vi "Circular Buffer(2D Wfm with Attributes).vi"(7 "Buffer Size":T3, 8 "error in (no error)":errorcluster, 9 "Read Size":i32, 10 "Operation":T1, 11 "Data In":waveform(dbl)[](array[waveform])) -> (0 "error out":errorcluster, 1 "Elements Remaining":i32, 2 "Buffer Status":T2, 3 "Data Out":waveform(dbl)[](array[waveform]))   [LabVIEW 2016, in "Circular Buffer.lvlib"]
doc: "This VI implements a circular buffer which data can be written to and read from. There can only be one buffer per data type at once, but you can have multiple buffers of different types at the same time. For example, you can have a buffer of Wfm data types as well as I32s in the same VI. You cannot have two independent buffers of I32s."
uses:
  Circular Buffer.lvlib
  Controls/Circular Buffer Status.ctl
  Controls/Circular Buffer Operations.ctl
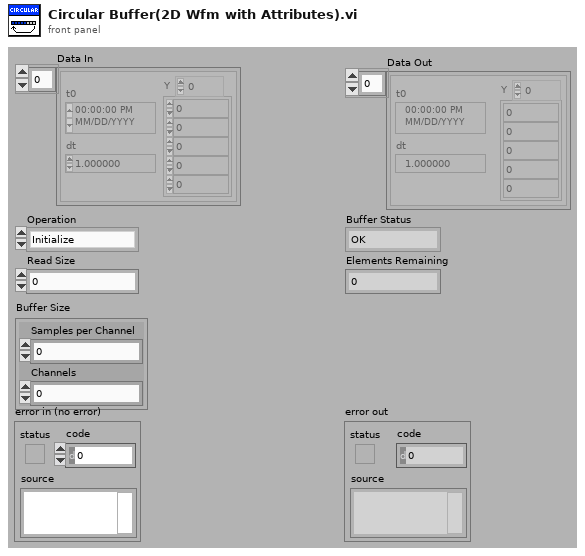
[diagram p1: front panel]
types:
  T1 = typedef "Circular Buffer.lvlib/Circular Buffer Operations.ctl" = enum16{"Initialize", "Get Backlog", "Write", "Read (continuous)", "Read (most recent)"}
  T2 = typedef "Circular Buffer.lvlib/Circular Buffer Status.ctl" = enum16{"OK", "Overflow", "Underflow"}
  T3 = cluster{"Samples per Channel":u32, "Channels":u32}
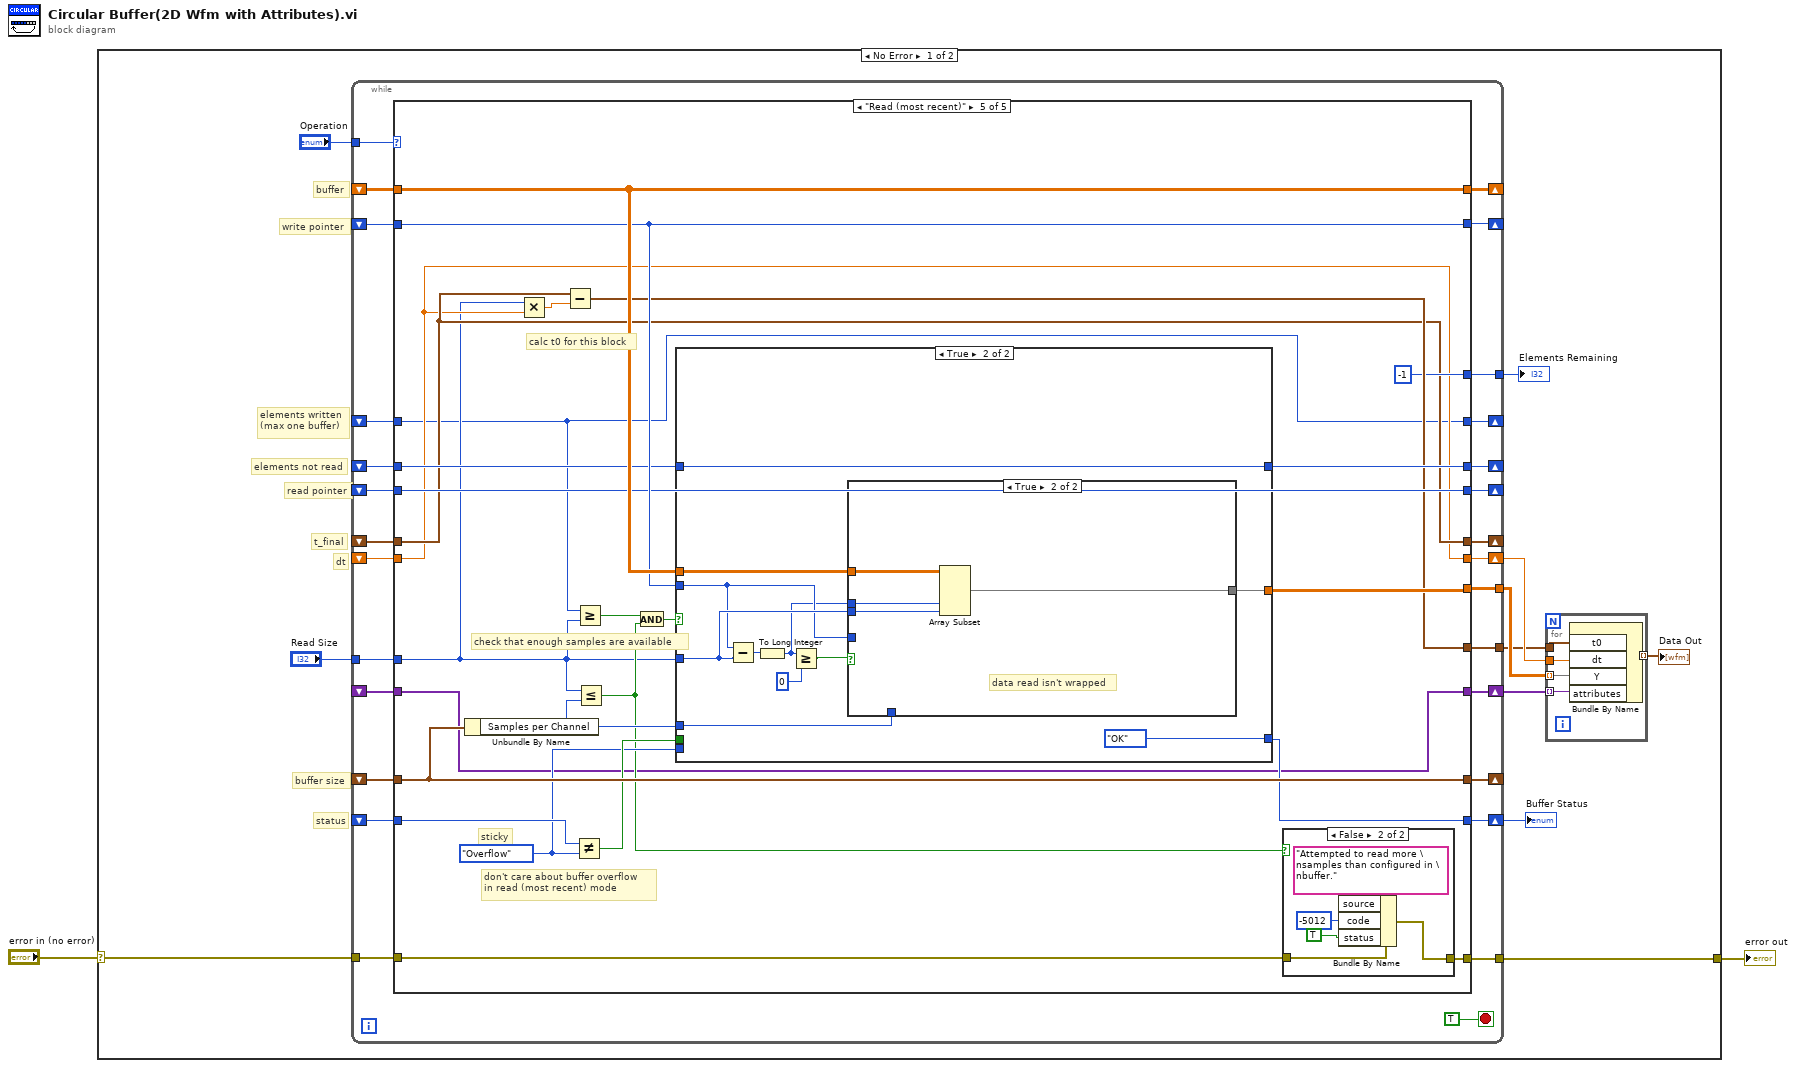
[diagram p0: block diagram]
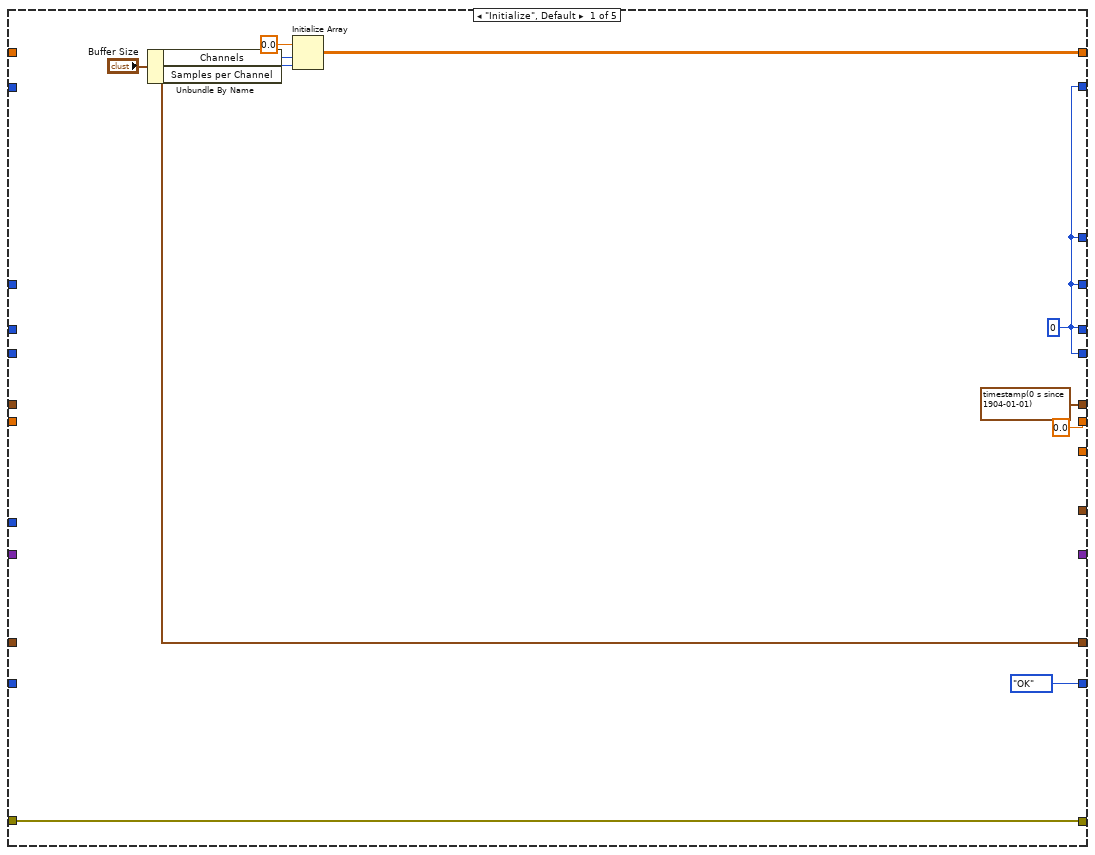
[diagram p2: hidden frame]
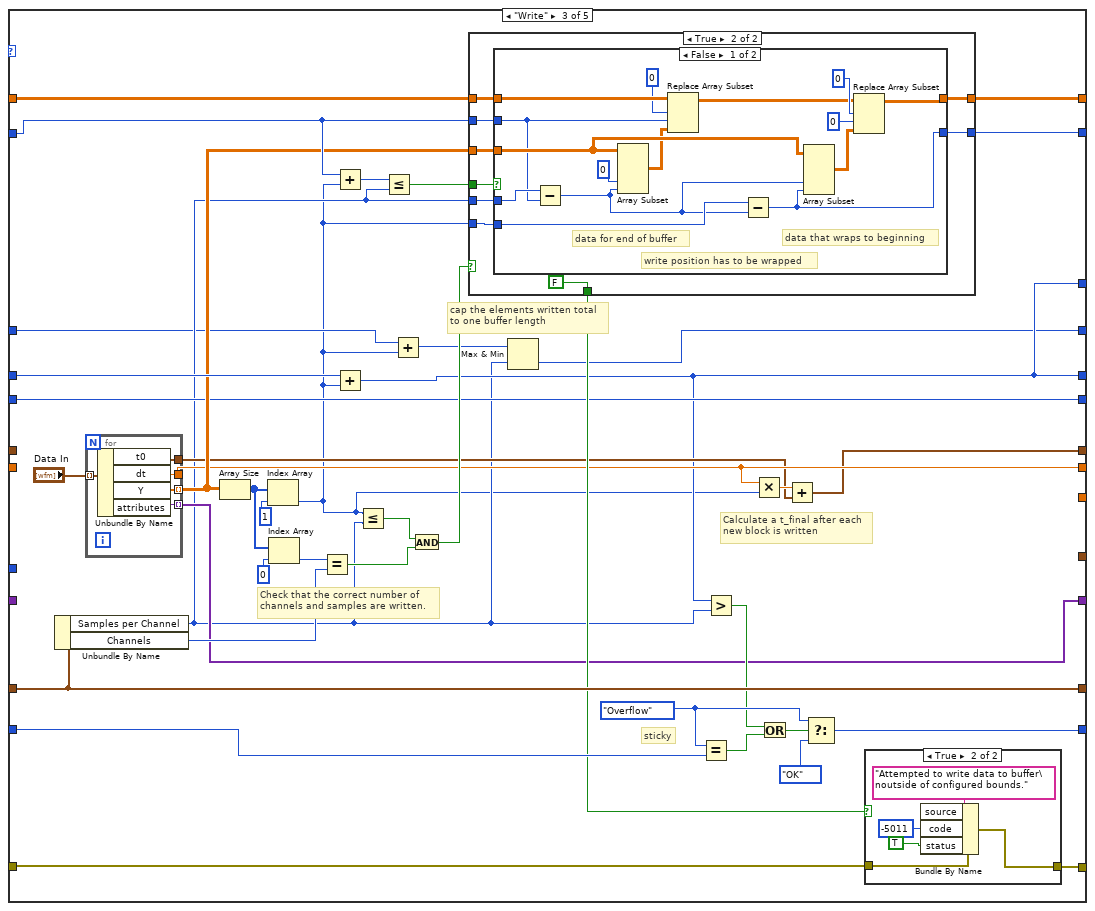
[diagram p4: hidden frame]
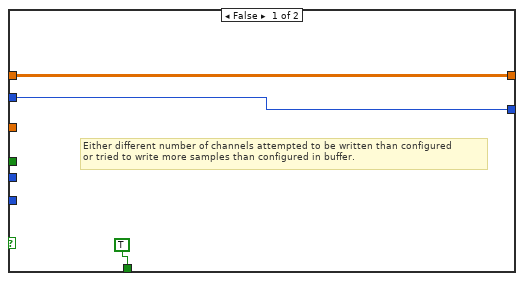
[diagram p6: hidden frame]
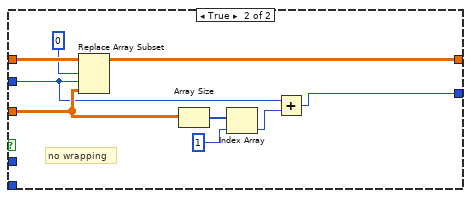
[diagram p7: hidden frame]
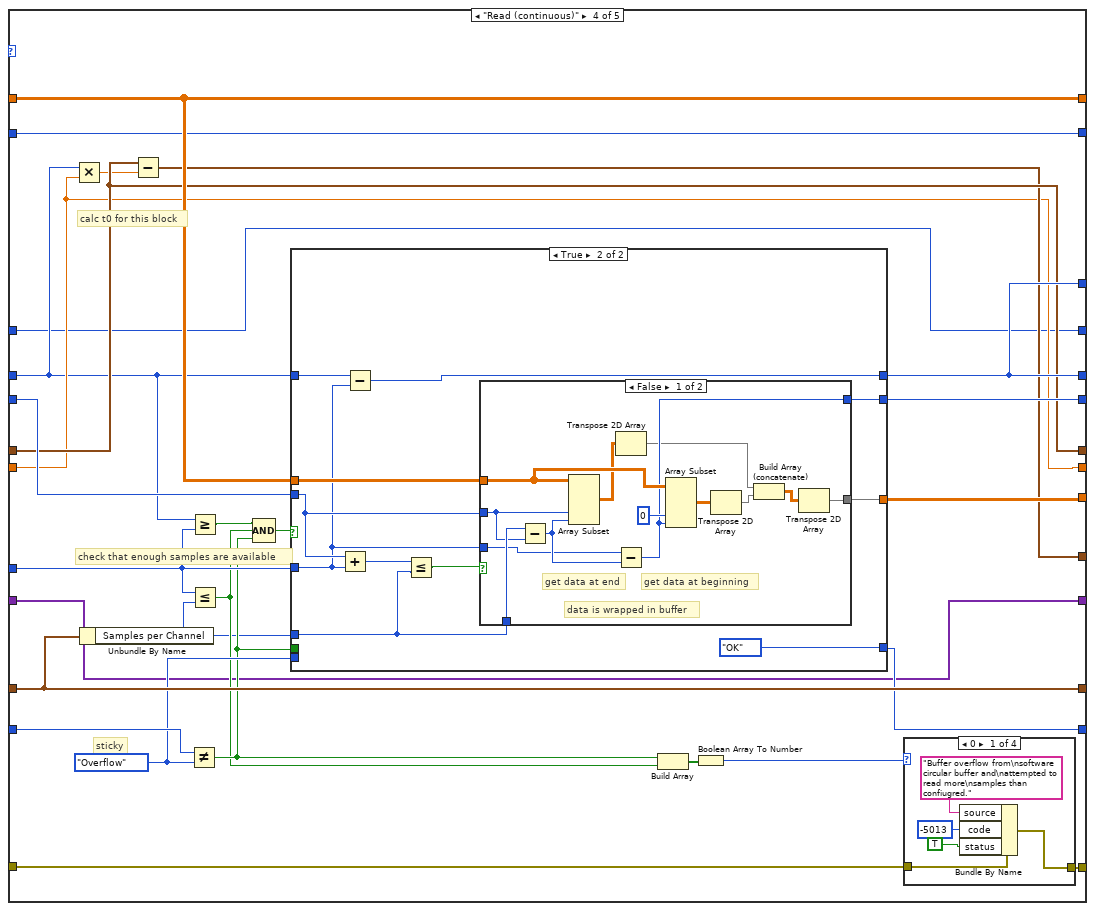
[diagram p8: hidden frame]
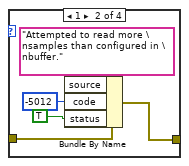
[diagram p9: hidden frame]
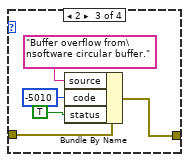
[diagram p10: hidden frame]
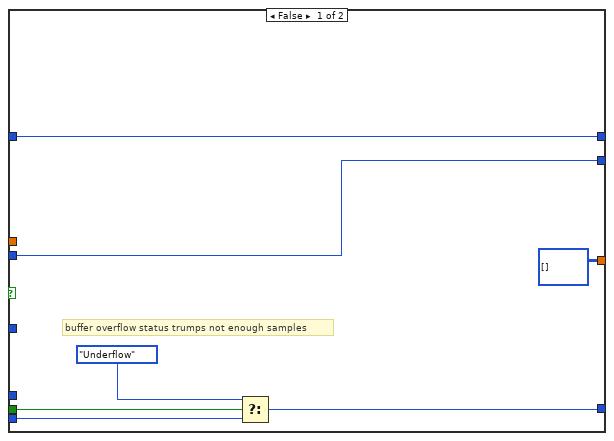
[diagram p12: hidden frame]
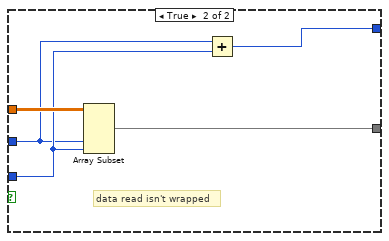
[diagram p13: hidden frame]
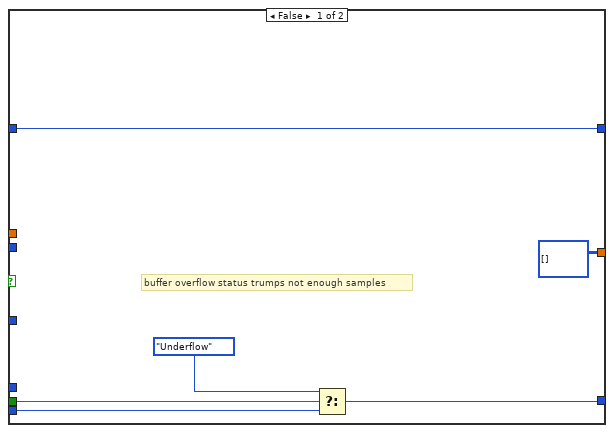
[diagram p15: hidden frame]
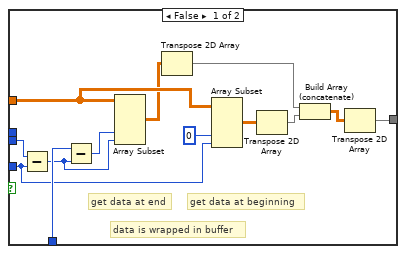
[diagram p16: hidden frame]
diagram:
  n1 = case shown="No Error" "error in (no error)" {
    selector: "error in (no error)" -> [w10 w298]
    tunnel: [w9 w298] -> w1
    frame No Error {
      # "elements written\n(max one buffer)"
      # "dt"
      # "t_final"
      # "write pointer"
      # "status"
      # "buffer size"
      # "read pointer"
      # "elements not read"
      # "buffer"
      n2 = while {
        tunnel: "Operation" -> [w45]
        shift-right: [w44] -> _
        shift-left: _ -> [w41]
        shift-right: [w43] -> _
        shift-left: _ -> [w40]
        shift-right: [w42] -> _
        shift-left: _ -> [w37]
        shift-right: [w39] -> _
        shift-left: _ -> [w38]
        tunnel: "Read Size" -> [w36]
        shift-right: [w35] -> w12
        shift-left: _ -> [w34]
        tunnel: [w33] -> w7
        tunnel: [w32] -> w9
        tunnel: w10 -> [w31]
        shift-right: [w30] -> _
        shift-left: _ -> [w29]
        shift-right: [w28] -> _
        shift-left: _ -> [w26]
        shift-right: [w27] -> w6
        shift-left: _ -> [w25]
        tunnel: [w24] -> w5
        tunnel: [w23] -> w4
        shift-right: [w22] -> w3
        shift-left: _ -> [w21]
        shift-right: [w19] -> _
        shift-left: _ -> [w20]
        stop <- TRUE stop-if-true
        n3 = case shown="\"Read (most recent)\"" w45 {
          tunnel: [w55 w65 w83 w180 w257] -> w44
          tunnel: [w47 w58 w71 w161 w252] -> w43
          tunnel: [w47 w60 w78 w163 w248] -> w42
          tunnel: w41 -> [_ w65 w82 w180 w257]
          tunnel: w40 -> [_ w58 w97 w156 w239]
          tunnel: ["Buffer Size" w59 w106 w179 w256] -> w39
          tunnel: w38 -> [_ w59 w106 w179 w256]
          tunnel: w37 -> [_ w60 w78 w176 w248]
          tunnel: w36 -> [_ _ _ w171 w236]
          tunnel: [Circular_Buffer_Status."OK" ("status") w64 w105 w175 w251] -> w35
          tunnel: w34 -> [_ w64 w102 w178 w255]
          tunnel: [_ _ _ w172 w250] -> w33
          tunnel: [w50 w66 w91 w174 w246] -> w32
          tunnel: w31 -> [w50 w66 w90 w173 w247]
          tunnel: [w47 w61 w79 w164 w249] -> w30
          tunnel: w29 -> [_ w61 w94 w164 w249]
          tunnel: [timestamp(0 s since 1904-01-01) ("t0") w63 w74 w160 w238] -> w28
          tunnel: [0.0 ("dt") w62 w76 w157 w237] -> w27
          tunnel: w26 -> [_ w63 _ w160 w238]
          tunnel: w25 -> [_ w62 _ w157 w237]
          tunnel: [_ _ _ w159 w241] -> w24
          tunnel: [w47 w58 w71 w161 -1] -> w23
          tunnel: [_ _ w73 w155 w234] -> w22
          tunnel: w21 -> [_ _ _ w155 w234]
          tunnel: w20 -> [_ w57 w69 w154 w233]
          tunnel: [w47 w57 w68 w154 w233] -> w19
          frame "Initialize", Default {
            w47 = 0 ("dimension size 2")
            n4 = Unbundle By Name("Buffer Size") -> ("Channels"=w52:u32, "Samples per Channel"=w51:u32)
            n5 = Initialize Array(0.0 ("element"), w52, w51) -> (w55:dbl[][])
          }
          frame "Get Backlog" {
          }
          frame "Write" {
            w101 = Circular_Buffer_Status."Overflow" ("status")
            # "cap the elements written total\nto one buffer length"
            # "Calculate a t_final after each\nnew block is written"
            # "Check that the correct number of\nchannels and samples are written."
            # "sticky"
            n6 = Unbundle By Name(w106) -> ("Samples per Channel"=w70:u32, "Channels"=w87:u32)
            n7 = for {
              tunnel: "Data In" -> [w111] mode=indexing
              tunnel: [w110] -> w80 mode=indexing
              tunnel: [w109] -> w76
              tunnel: [w108] -> w75
              tunnel: [w107] -> w73 mode=indexing
              n8 = Unbundle By Name(w111) -> ("t0"=w108:timestamp, "dt"=w109:dbl, "Y"=w110:dbl[], "attributes"=w107:variant)
            }
            n9 = Array Size(array=w80) -> (size(s)=w93:i32[])
            n10 = Index Array(array=w93, index=1) -> (element=w67:i32)
            n11 = Index Array(array=w93, index=0) -> (element=w88:i32)
            n12 = Equal?(x=w88, y=w87) -> (x = y?=w85:bool)
            n13 = Add(x=w94, y=w67) -> (x+y=w96:u32)
            n14 = Add(x=w97, y=w67) -> (x+y=w71:i32)
            n15 = Less Or Equal?(x=w67, y=w70) -> (x <= y?=w86:bool)
            n16 = Less Or Equal?(x=w96, y=w70) -> (x <= y?=w95:bool)
            n17 = Add(x=w69, y=w67) -> (x+y=w72:u32)
            n18 = And(x=w86, y=w85) -> (x .and. y?=w84:bool)
            n19 = case shown="True" w84 {
              tunnel: [w120 w129] -> w83
              tunnel: w95 -> [_ w128]
              tunnel: [w119 w127] -> w79
              tunnel: w94 -> [w119 w126]
              tunnel: w82 -> [w120 w125]
              tunnel: w80 -> [_ w124]
              tunnel: w67 -> [_ w123]
              tunnel: w70 -> [_ w122]
              tunnel: [TRUE FALSE] -> w89
              frame False {
                # "Either different number of channels attempted to be written than configured\nor tried to write more samples than configured in buffer."
              }
              frame True {
                n20 = case shown="False" w128 {
                  tunnel: w125 -> [w144 w153]
                  tunnel: [w139 w151] -> w129
                  tunnel: w126 -> [w133 w146]
                  tunnel: w124 -> [w137 w148]
                  tunnel: w122 -> [w134 _]
                  tunnel: w123 -> [w136 _]
                  tunnel: [w135 w145] -> w127
                  frame False {
                    # "data that wraps to beginning"
                    # "data for end of buffer"
                    # "write position has to be wrapped"
                    n21 = Subtract(x=w134, y=w133) -> (x-y=w132:u32)
                    n22 = Array Subset(array=w137, index (col)=0 ("index"), length (col)=w132) -> (w131:dbl[][])  [unwired: 2 in]
                    n23 = Replace Array Subset(array=w144, new element=w131, index (row)=0, index (col)=w133) -> (w140:dbl[][])
                    n24 = Subtract(x=w136, y=w132) -> (x-y=w135:u32)
                    n25 = Array Subset(array=w137, index (col)=w132, length (col)=w135) -> (w142:dbl[][])  [unwired: 2 in]
                    n26 = Replace Array Subset(array=w140, new element=w142, index (row)=0, index (col)=0 ("disabled index (col)")) -> (w139:dbl[][])
                  }
                  frame True {
                    # "no wrapping"
                    n27 = Replace Array Subset(array=w153, new element=w148, index (row)=0 ("disabled index (col)"), index (col)=w146) -> (w151:dbl[][])
                    n28 = Array Size(array=w148) -> (size(s)=w150:i32[])
                    n29 = Index Array(array=w150, index=1) -> (element=w147:i32)
                    n30 = Add(x=w146, y=w147) -> (x+y=w145:u32)
                  }
                }
              }
            }
            n31 = Max & Min(x=w72, y=w70) -> (min(x,y)=w68:u32)  [unwired: 1 out]
            n32 = Equal?(x=w101, y=w102) -> (x = y?=w104:bool)
            n33 = Greater?(x=w71, y=w70) -> (0:w99:bool)
            n34 = Multiply(x=w76, y=w67) -> (x*y=w77:dbl)
            n35 = Or(x=w99, y=w104) -> (x .or. y?=w103:bool)
            n36 = Add(x=w77, y=w75) -> (x+y=w74:timestamp)
            n37 = Select(t=w101, s=w103, f=Circular_Buffer_Status."OK" ("status")) -> (s? t:f=w105:T2)
            n38 = case shown="True" w89 {
              tunnel: w90 -> [w112 w117]
              tunnel: [w112 w116] -> w91
              frame False {
              }
              frame True {
                n39 = Bundle By Name(cluster=w117, "source"="Attempted to write data to buffer\noutside of configured bounds.", "code"=-5011, "status"=TRUE) -> (w116:errorcluster)
              }
            }
          }
          frame "Read (continuous)" {
            w177 = Circular_Buffer_Status."Overflow" ("status")
            # "calc t0 for this block"
            # "check that enough samples are available"
            # "sticky"
            n40 = Multiply(x=w156, y=w157) -> (x*y=w158:dbl)
            n41 = Unbundle By Name(w179) -> ("Samples per Channel"=w162:u32)
            n42 = Subtract(x=w160, y=w158) -> (x-y=w159:timestamp)
            n43 = Not Equal?(x=w178, y=w177) -> (x != y?=w168:bool)
            n44 = Greater Or Equal?(x=w156, y=w171) -> (x >= y?=w170:bool)
            n45 = Less Or Equal?(x=w171, y=w162) -> (x <= y?=w167:bool)
            n46 = Compound Arithmetic op=AND(w170, w167, w168) -> (w169:bool)
            n47 = case shown="True" w169 {
              tunnel: w176 -> [w198 w207]
              tunnel: w180 -> [_ w213]
              tunnel: w171 -> [_ w205]
              tunnel: w162 -> [_ w208]
              tunnel: [w202 Circular_Buffer_Status."OK" ("status")] -> w175
              tunnel: w168 -> [w203 _]
              tunnel: w177 -> [w201 _]
              tunnel: w156 -> [w199 w206]
              tunnel: [w199 w204] -> w161
              tunnel: [w198 w209] -> w163
              tunnel: [i32[][] [] w210] -> w172
              frame False {
                # "buffer overflow status trumps not enough samples"
                n48 = Select(t=Circular_Buffer_Status."Underflow" ("status"), s=w203, f=w201) -> (s? t:f=w202:T2)
              }
              frame True {
                n49 = Add(x=w207, y=w205) -> (x+y=w212:u32)
                n50 = Subtract(x=w206, y=w205) -> (x-y=w204:i32)
                n51 = Less Or Equal?(x=w212, y=w208) -> (x <= y?=w211:bool)
                n52 = case shown="False" w211 {
                  tunnel: w213 -> [w226 w232]
                  tunnel: w207 -> [w222 w229]
                  tunnel: w205 -> [w215 w230]
                  tunnel: [w217 w231] -> w210
                  tunnel: [w223 w228] -> w209
                  tunnel: w208 -> [w227 _]
                  frame False {
                    # "get data at beginning"
                    # "get data at end"
                    # "data is wrapped in buffer"
                    n53 = Subtract(x=w227, y=w222) -> (x-y=w224:u32)
                    n54 = Array Subset(array=w226, index (col)=w222, length (col)=w224) -> (w221:dbl[][])  [unwired: 2 in]
                    n55 = Transpose 2D Array(2D array=w221) -> (transposed array=w219:dbl[][])
                    n56 = Subtract(x=w215, y=w224) -> (x-y=w223:u32)
                    n57 = Array Subset(array=w226, index (col)=0 ("index"), length (col)=w223) -> (w220:dbl[][])  [unwired: 2 in]
                    n58 = Transpose 2D Array(2D array=w220) -> (transposed array=w218:dbl[][])
                    n59 = Build Array (concatenate)(w219, w218) -> (w216:dbl[][])
                    n60 = Transpose 2D Array(2D array=w216) -> (transposed array=w217:dbl[][])
                  }
                  frame True {
                    # "data read isn't wrapped"
                    n61 = Array Subset(array=w232, index (col)=w229, length (col)=w230) -> (w231:dbl[][])  [unwired: 2 in]
                    n62 = Add(x=w229, y=w230) -> (x+y=w228:u32)
                  }
                }
              }
            }
            n63 = Build Array(w168, w167) -> (w166:bool[])
            n64 = Boolean Array To Number(Boolean array=w166) -> (number=w165:u32)
            n65 = case shown="0" w165 {
              tunnel: w173 -> [w185 w190 w195 w196]
              tunnel: [w184 w189 w194 w196] -> w174
              frame 0 {
                n66 = Bundle By Name(cluster=w185, "source"="Buffer overflow from\nsoftware circular buffer and\nattempted to read more\nsamples than confiugred.", "code"=-5013, "status"=TRUE) -> (w184:errorcluster)
              }
              frame 1 {
                n67 = Bundle By Name(cluster=w190, "source"="Attempted to read more \nsamples than configured in \nbuffer.", "code"=-5012, "status"=TRUE) -> (w189:errorcluster)
              }
              frame 2 {
                n68 = Bundle By Name(cluster=w195, "source"="Buffer overflow from\nsoftware circular buffer.", "code"=-5010, "status"=TRUE) -> (w194:errorcluster)
              }
              frame 3, Default {
              }
            }
          }
          frame "Read (most recent)" {
            w253 = Circular_Buffer_Status."Overflow" ("status")
            # "calc t0 for this block"
            # "don't care about buffer overflow\nin read (most recent) mode"
            # "check that enough samples are available"
            # "sticky"
            n69 = Unbundle By Name(w256) -> ("Samples per Channel"=w245:u32)
            n70 = Multiply(x=w236, y=w237) -> (x*y=w235:dbl)
            n71 = Subtract(x=w238, y=w235) -> (x-y=w241:timestamp)
            n72 = Not Equal?(x=w255, y=w253) -> (x != y?=w254:bool)
            n73 = Greater Or Equal?(x=w233, y=w236) -> (x >= y?=w243:bool)
            n74 = Less Or Equal?(x=w236, y=w245) -> (x <= y?=w242:bool)
            n75 = And(x=w243, y=w242) -> (x .and. y?=w244:bool)
            n76 = case shown="True" w244 {
              tunnel: w249 -> [_ w272]
              tunnel: w257 -> [_ w278]
              tunnel: w236 -> [_ w274]
              tunnel: w245 -> [_ w275]
              tunnel: [w268 Circular_Buffer_Status."OK" ("status")] -> w251
              tunnel: w254 -> [w269 _]
              tunnel: w253 -> [w267 _]
              tunnel: w239 -> [w265 w279]
              tunnel: [w265 w279] -> w252
              tunnel: [i32[][] [] w276] -> w250
              frame False {
                # "buffer overflow status trumps not enough samples"
                n77 = Select(t=Circular_Buffer_Status."Underflow" ("status"), s=w269, f=w267) -> (s? t:f=w268:T2)
              }
              frame True {
                n78 = Subtract(x=w272, y=w274) -> (x-y=w270:u32)
                n79 = To Long Integer(number=w270) -> (32bit integer=w271:i32)
                n80 = Greater Or Equal?(x=w271, y=0) -> (x >= y?=w277:bool)
                n81 = case shown="True" w277 {
                  tunnel: w278 -> [w292 w297]
                  tunnel: [w286 w296] -> w276
                  tunnel: w275 -> [w293 _]
                  tunnel: w271 -> [_ w295]
                  tunnel: w274 -> [w284 w294]
                  tunnel: w272 -> [w281 _]
                  frame False {
                    # "get data at beginning"
                    # "get data at end"
                    # "data is wrapped in buffer"
                    n82 = Subtract(x=w284, y=w281) -> (x-y=w282:u32)
                    n83 = Subtract(x=w293, y=w282) -> (x-y=w283:u32)
                    n84 = Array Subset(array=w292, index (col)=w283, length (col)=w282) -> (w290:dbl[][])  [unwired: 2 in]
                    n85 = Transpose 2D Array(2D array=w290) -> (transposed array=w288:dbl[][])
                    n86 = Array Subset(array=w292, index (col)=0 ("index"), length (col)=w281) -> (w289:dbl[][])  [unwired: 2 in]
                    n87 = Transpose 2D Array(2D array=w289) -> (transposed array=w287:dbl[][])
                    n88 = Build Array (concatenate)(w288, w287) -> (w285:dbl[][])
                    n89 = Transpose 2D Array(2D array=w285) -> (transposed array=w286:dbl[][])
                  }
                  frame True {
                    # "data read isn't wrapped"
                    n90 = Array Subset(array=w297, index (col)=w295, length (col)=w294) -> (w296:dbl[][])  [unwired: 2 in]
                  }
                }
              }
            }
            n91 = case shown="False" w242 {
              tunnel: w247 -> [w258 w263]
              tunnel: [w258 w262] -> w246
              frame True {
              }
              frame False {
                n92 = Bundle By Name(cluster=w263, "source"="Attempted to read more \nsamples than configured in \nbuffer.", "code"=-5012, "status"=TRUE) -> (w262:errorcluster)
              }
            }
          }
        }
      }
      "Elements Remaining" <- w4
      "Buffer Status" <- w12
      n93 = for {
        tunnel: [w18] -> w8 mode=indexing
        tunnel: w7 -> [w17] mode=indexing
        tunnel: w6 -> [w16]
        tunnel: w5 -> [w15]
        tunnel: w3 -> [w14] mode=indexing
        n94 = Bundle By Name("t0"=w15, "dt"=w16, "Y"=w17, "attributes"=w14) -> (w18:waveform(dbl))  [unwired: 1 out]
      }
      "Data Out" <- w8
    }
    frame Error {
    }
  }
  "error out" <- w1
